vi "LoadArrayINI (SubVI).vi"(7 "Numeric":i32, 8 "error in (no error)":errorcluster, 9 "section":string, 10 "key":string, 11 "Refnum in":T1) -> (0 "error out":errorcluster, 2 "Array":dbl[](array[numeric]), 3 "Refnum out":T1)   [LabVIEW 2017]
uses:
  <vilib>/Utility/config.llb/Config Data RefNum.ctl
  <vilib>/Utility/config.llb/Read Key (Double).vi
  <vilib>/Utility/config.llb/NI_LVConfig.lvlib
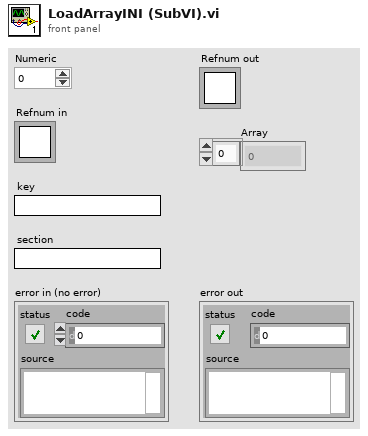
[diagram p1: front panel]
types:
  T1 = typedef "NI_LVConfig.lvlib/Config Data RefNum.ctl" = refnum<k1>
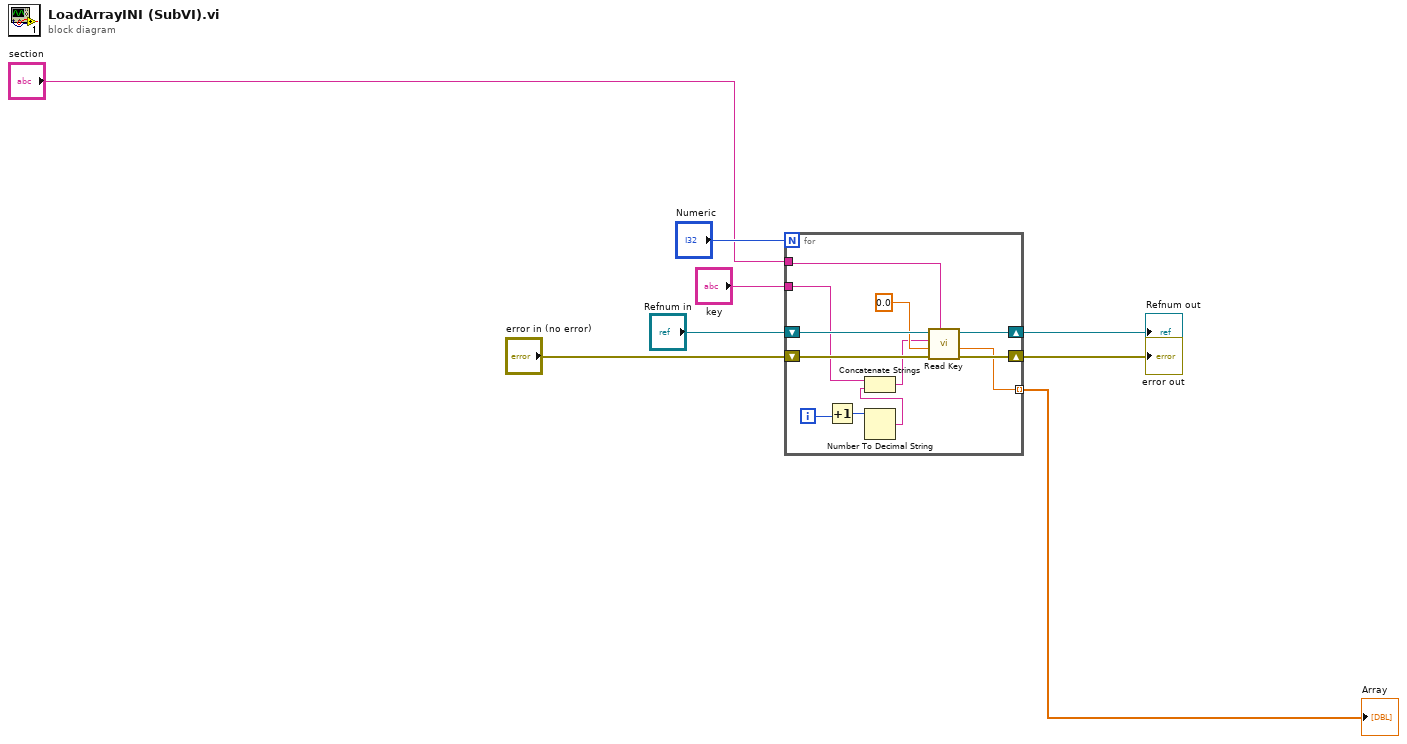
[diagram p0: block diagram]
diagram:
  n1 = for {
    N: "Numeric" -> [_]
    tunnel: "section" -> [w15]
    shift-right: [w17] -> w6
    shift-left: "Refnum in" -> [w20]
    shift-right: [w18] -> w7
    shift-left: "error in (no error)" -> [w19]
    tunnel: [w14] -> w5 mode=indexing
    tunnel: "key" -> [w9]
    i -> [w13]
    n2 = Increment(x=w13) -> (x+1=w12:i32)
    n3 = Number To Decimal String(number=w12) -> (decimal integer string=w11:string)  [unwired: 1 in]
    n4 = Concatenate Strings(w9, w11) -> (w10:string)
    n5 = call-poly <vilib>:"Read Key.vi"("section"=w15, "error in (no error)"=w19, "default value"=0.0, "key"=w10, "refnum"=w20) -> ("error out"=w18:errorcluster, "value"=w14:dbl, "refnum out"=w17:T1)  [unwired: 3 in, 1 out]
  }
  "error out" <- w7
  "Refnum out" <- w6
  "Array" <- w5
